vi "Graph (SubVI).vi"(9 "MeasChanel":u32[](array[numeric]), 10 "Parameters":T4={"UNDT_Type_signal"=enum."РЧ сигнал", "ФНЧ"=TRUE, "UNDT_Mean"=1, "IIR filter"={"Topology"=enum."Off", "Type"=enum."Bandpass", "Order"=4, "Lower Fc"=200000.0, "Upper Fc"=10000000.0, "PB Ripple"=1.0, "SB Attenuation"=60.0}, "ZeroDimension"=4000, "ТипДетектора"=enum."Оконный детектор", "FilterCor"={"HPFFilterNum"=enum."HPF_OFF", "LPFBode"=[], "HPFBode"=[], "EnableFilterСorrect"=FALSE, "LPF_Filter"=enum."14 МГц"}, "MeasControl"={"approx freq"=-1.0, "search (+/- % of Fsampl.)"=1.0, "start, duration"={"start samples/time"=-1.0, "duration"=0.0, "EnableSubset"=FALSE}, "averaging type"=enum."Linear", "window"=enum."Rectangular (none)", "hysteresis"=0.0, "level"=0.0}} {"MeasControl"."level" format="%.2p"; "MeasControl"."hysteresis" format="%.2p"; "MeasControl"."start, duration"."duration" format="%0.2f"; "MeasControl"."start, duration"."start samples/time" format="%0.2f"; "MeasControl"."search (+/- % of Fsampl.)" format="%#_13g"; "IIR filter"."PB Ripple" format="%0.2f"; "IIR filter"."SB Attenuation" format="%0.2f"; "IIR filter"."Lower Fc" format="%0.2p"; "IIR filter"."Upper Fc" format="%0.2p"; "UNDT_Mean" min=0 max=32 step=4}, 11 "DataIn":T1 {"UNDT_Cluster"."Gain Coeff" format="%#_6e"; "UNDT_Cluster"."Reserve 1" format="%02x"; "UNDT_Cluster"."Mux TX/RX" format="%02x"; "UNDT_Cluster"."ScanDelay" format="%02x"; "UNDT_Cluster"."PacketCounter" format="%08x"; "UNDT_Cluster"."SamplingInterval" format="%#_6e"; "UNDT_Cluster"."Lose Packet" format="%08x"; "UNDT_Cluster"."EncodersParam2" format="%016x"; "UNDT_Cluster"."EncodersParam1" format="%016x"; "UNDT_Cluster"."CRC 8" format="%02x"; "UNDT_Cluster"."N chanel" format="%02x"; "UNDT_Cluster"."N tick" format="%02x"; "UNDT_Cluster"."Ncycle" format="%04x"; "UNDT_Cluster"."FrameFormatVersion" format="%02x"; "UNDT_Cluster"."MagicWord" format="%.0x"}) -> (2 "Meas":T3 {"FFT amplitude mean" format="%.2p"; "DC" format="%0.2p"; "time trig 2" format="%0.2p"; "time trig" format="%0.2p"; "detected frequency 2" format="%.2p"; "way sensor 2" format="%.2p"; "way sensor 1" format="%.2p"; "detected frequency" format="%.2p"; "RMS" format="%0.2p"; "amplitude" format="%.2p"; "FFT amplitude" format="%.2p"}, 3 "Filtered X":dbl[](array[numeric]))   [LabVIEW 2017]
uses:
  Control_EU/UNDT_Graph (Type).ctl
  Control_EU/MeasControl2.ctl
  Control_EU/MeasControl.ctl
  Control_EU/DataCluster.ctl
  Control_EU/UNDT_ClusterPackRevers (Type).ctl
  <vilib>/Analysis/baseanly.llb/Mean (DBL).vi
  <vilib>/Analysis/NI_AALBase.lvlib
panel:
  out "Boolean":bool
  out "N tick":u8
  out "detected frequency":dbl
  out "FilterCorCoef":dbl
  out "MeanSizeLast":i32=8
  out "Tick 63":dbl[][](array[numeric])
  out "Tick 62":dbl[][](array[numeric])
  out "Tick 61":dbl[][](array[numeric])
  out "Tick 60":dbl[][](array[numeric])
  out "Tick 59":dbl[][](array[numeric])
  out "Tick 58":dbl[][](array[numeric])
  out "Tick 57":dbl[][](array[numeric])
  out "Tick 56":dbl[][](array[numeric])
  out "Tick 55":dbl[][](array[numeric])
  out "Tick 54":dbl[][](array[numeric])
  out "Tick 53":dbl[][](array[numeric])
  out "Tick 52":dbl[][](array[numeric])
  out "Tick 51":dbl[][](array[numeric])
  out "Tick 50":dbl[][](array[numeric])
  out "Tick 49":dbl[][](array[numeric])
  out "Tick 48":dbl[][](array[numeric])
  out "Tick 47":dbl[][](array[numeric])
  out "Tick 46":dbl[][](array[numeric])
  out "Tick 45":dbl[][](array[numeric])
  out "Tick 44":dbl[][](array[numeric])
  out "Tick 43":dbl[][](array[numeric])
  out "Tick 42":dbl[][](array[numeric])
  out "Tick 41":dbl[][](array[numeric])
  out "Tick 40":dbl[][](array[numeric])
  out "Tick 39":dbl[][](array[numeric])
  out "Tick 38":dbl[][](array[numeric])
  out "Tick 37":dbl[][](array[numeric])
  out "Tick 36":dbl[][](array[numeric])
  out "Tick 35":dbl[][](array[numeric])
  out "Tick 34":dbl[][](array[numeric])
  out "Tick 33":dbl[][](array[numeric])
  out "Tick 32":dbl[][](array[numeric])
  out "Tick 31":dbl[][](array[numeric])
  out "Tick 30":dbl[][](array[numeric])
  out "Tick 29":dbl[][](array[numeric])
  out "Tick 28":dbl[][](array[numeric])
  out "Tick 27":dbl[][](array[numeric])
  out "Tick 26":dbl[][](array[numeric])
  out "Tick 25":dbl[][](array[numeric])
  out "Tick 24":dbl[][](array[numeric])
  out "Tick 23":dbl[][](array[numeric])
  out "Tick 22":dbl[][](array[numeric])
  out "Tick 21":dbl[][](array[numeric])
  out "Tick 20":dbl[][](array[numeric])
  out "Tick 19":dbl[][](array[numeric])
  out "Tick 18":dbl[][](array[numeric])
  out "Tick 17":dbl[][](array[numeric])
  out "Tick 16":dbl[][](array[numeric])
  out "Tick 15":dbl[][](array[numeric])
  out "Tick 14":dbl[][](array[numeric])
  out "Tick 13":dbl[][](array[numeric])
  out "Tick 12":dbl[][](array[numeric])
  out "Tick 11":dbl[][](array[numeric])
  out "Tick 10":dbl[][](array[numeric])
  out "Tick 9":dbl[][](array[numeric])
  out "Tick 8":dbl[][](array[numeric])
  out "Tick 7":dbl[][](array[numeric])
  out "Tick 6":dbl[][](array[numeric])
  out "Tick 5":dbl[][](array[numeric])
  out "Tick 4":dbl[][](array[numeric])
  out "Tick 3":dbl[][](array[numeric])
  out "Tick 2":dbl[][](array[numeric])
  out "Tick 1":dbl[][](array[numeric])
  out "Tick 0":dbl[][](array[numeric])
  out "MeanSize":i32=8
  out "Index Aarray":i32[](array[numeric])
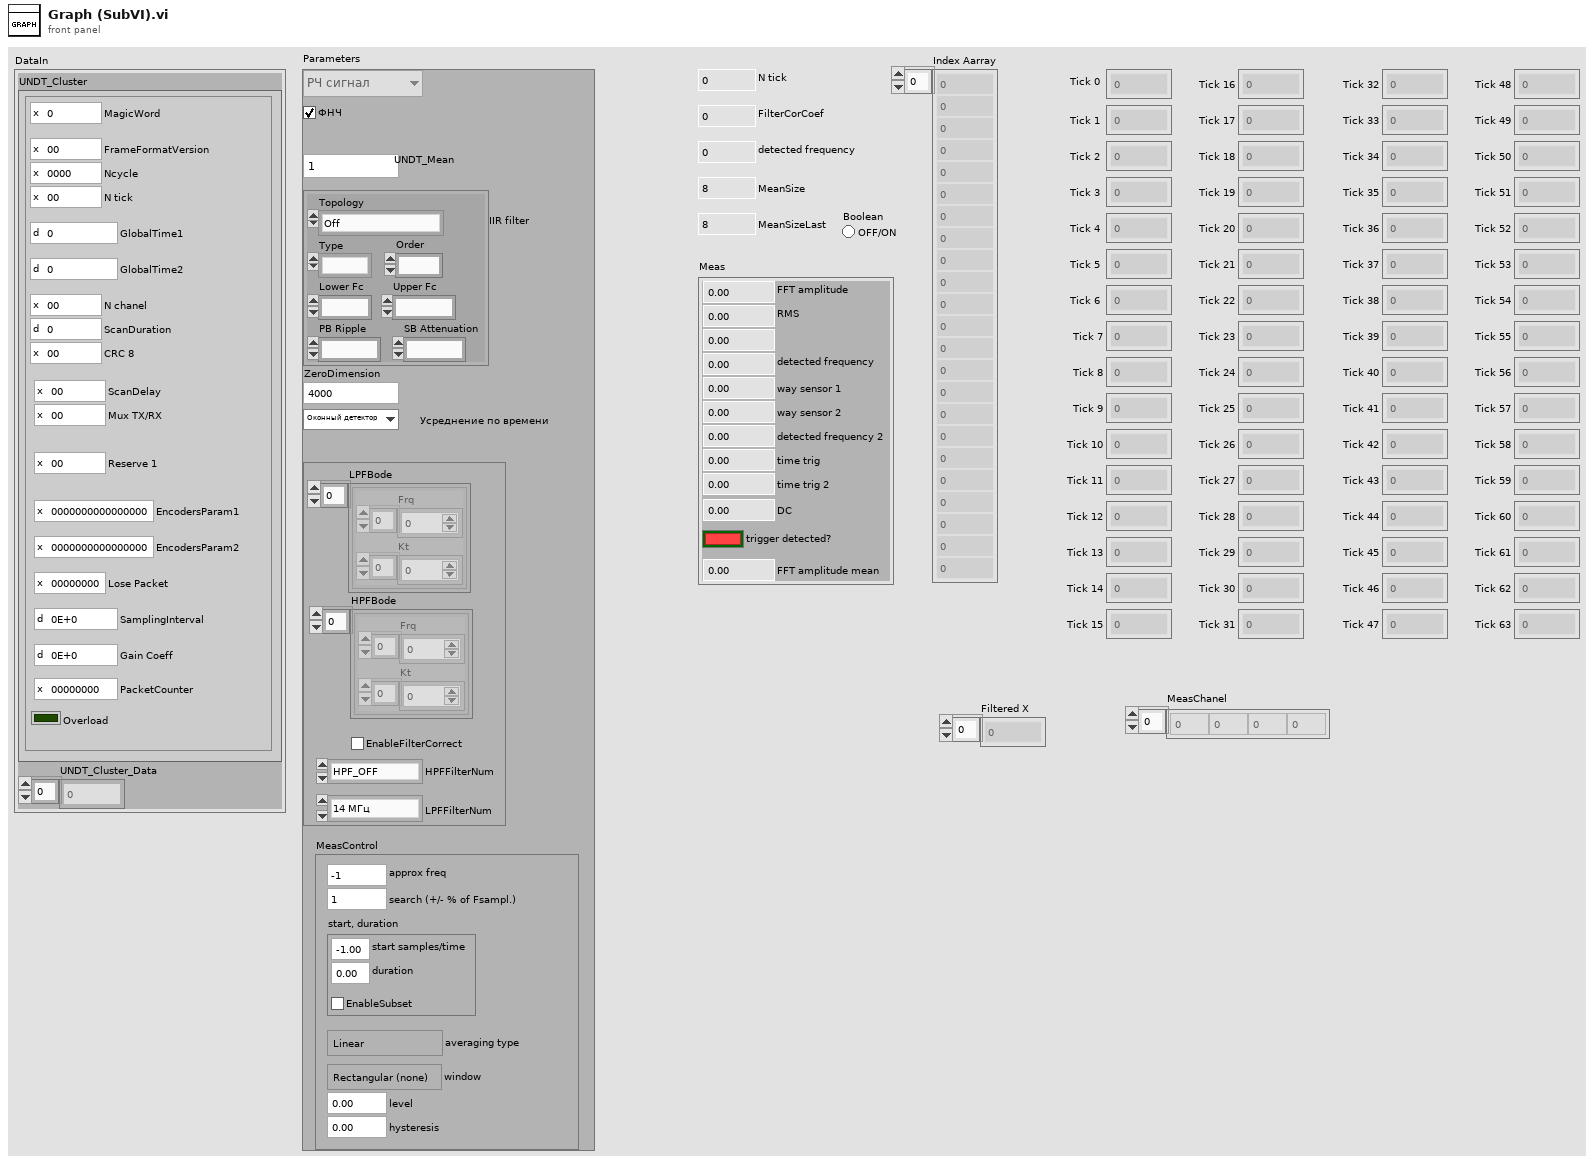
[diagram p1: front panel]
types:
  T1 = typedef "DataCluster.ctl" = cluster{"UNDT_Cluster":T2, "UNDT_Cluster_Data":dbl[]}
  T2 = typedef "UNDT_ClusterPackRevers (Type).ctl" = cluster{"PacketCounter":u32, "Gain Coeff":sgl, "SamplingInterval":sgl, "Lose Packet":u32, "EncodersParam2":u64, "EncodersParam1":u64, "Reserve 1":u8, "Mux TX/RX":u8, "ScanDelay":u16, "CRC 8":u8, "ScanDuration":u16, "N chanel":u8, "GlobalTime2":u32, "GlobalTime1":u32, "N tick":u8, "Ncycle":u16, "FrameFormatVersion":u8, "MagicWord":u32, "Overload":bool}
  T3 = typedef "MeasControl.ctl" = cluster{"FFT amplitude":dbl, "amplitude":dbl, "RMS":dbl, "detected frequency":dbl, "way sensor 1":ext, "way sensor 2":ext, "detected frequency 2":dbl, "time trig":dbl, "time trig 2":dbl, "DC":dbl, "trigger detected?":bool, "FFT amplitude mean":dbl}
  T4 = typedef "UNDT_Graph (Type).ctl" = cluster{"UNDT_Type_signal":enum16{"РЧ сигнал", "Детект. полное", "Положит.", "Отрицат."}, "ФНЧ":bool, "UNDT_Mean":i32, "IIR filter":cluster{"Topology":enum16{"Off", "Butterworth", "Chebyshev", "Inverse Chebyshev", "Elliptic", "Bessel"}, "Type":enum16{"Lowpass", "Highpass", "Bandpass", "Bandstop"}, "Order":i32, "Lower Fc":dbl, "Upper Fc":dbl, "PB Ripple":dbl, "SB Attenuation":dbl}, "ZeroDimension":i32, "ТипДетектора":enum16{"Оконный детектор", "Гильберт"}, "FilterCor":cluster{"HPFFilterNum":enum16{"HPF_OFF", "1", "2", "3", "4", "5", "6", "7", "8", "9", "10"}, "LPFBode":cluster{"Frq":dbl[], "Kt":dbl[]}[], "HPFBode":cluster{"Frq":dbl[], "Kt":dbl[]}[], "EnableFilterСorrect":bool, "LPF_Filter":enum16{"14 МГц", "10 МГц", "7.5 МГц", "Выкл."}}, "MeasControl":T5}
  T5 = typedef "MeasControl2.ctl" = cluster{"approx freq":dbl, "search (+/- % of Fsampl.)":dbl, "start, duration":cluster{"start samples/time":dbl, "duration":dbl, "EnableSubset":bool}, "averaging type":enum16{"Linear", "Exponential"}, "window":enum16{"Rectangular (none)", "Hanning", "Low side lobe"}, "hysteresis":dbl, "level":dbl}
  T6 = enum16{"РЧ сигнал", "Детект. полное", "Положит.", "Отрицат."}
  T7 = cluster{"Topology":enum16{"Off", "Butterworth", "Chebyshev", "Inverse Chebyshev", "Elliptic", "Bessel"}, "Type":enum16{"Lowpass", "Highpass", "Bandpass", "Bandstop"}, "Order":i32, "Lower Fc":dbl, "Upper Fc":dbl, "PB Ripple":dbl, "SB Attenuation":dbl}
  T8 = cluster{"HPFFilterNum":enum16{"HPF_OFF", "1", "2", "3", "4", "5", "6", "7", "8", "9", "10"}, "LPFBode":cluster{"Frq":dbl[], "Kt":dbl[]}[], "HPFBode":cluster{"Frq":dbl[], "Kt":dbl[]}[], "EnableFilterСorrect":bool, "LPF_Filter":enum16{"14 МГц", "10 МГц", "7.5 МГц", "Выкл."}}
  T9 = enum16{"HPF_OFF", "1", "2", "3", "4", "5", "6", "7", "8", "9", "10"}
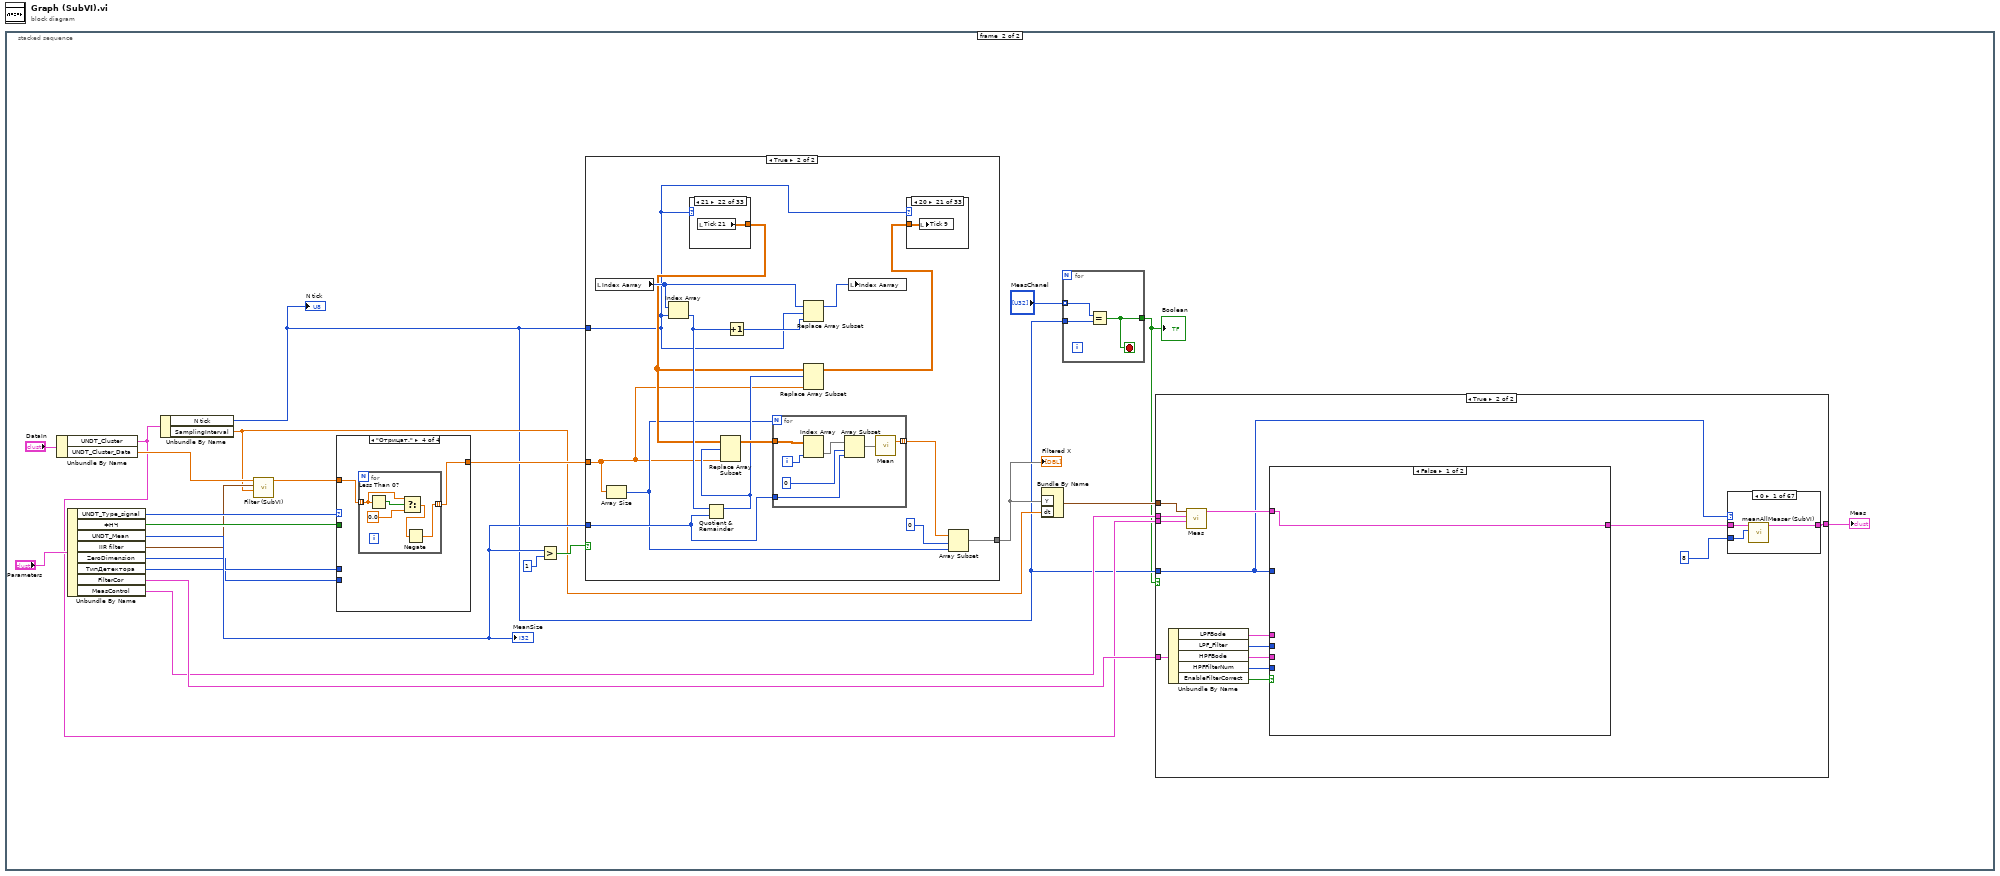
[diagram p0: block diagram]
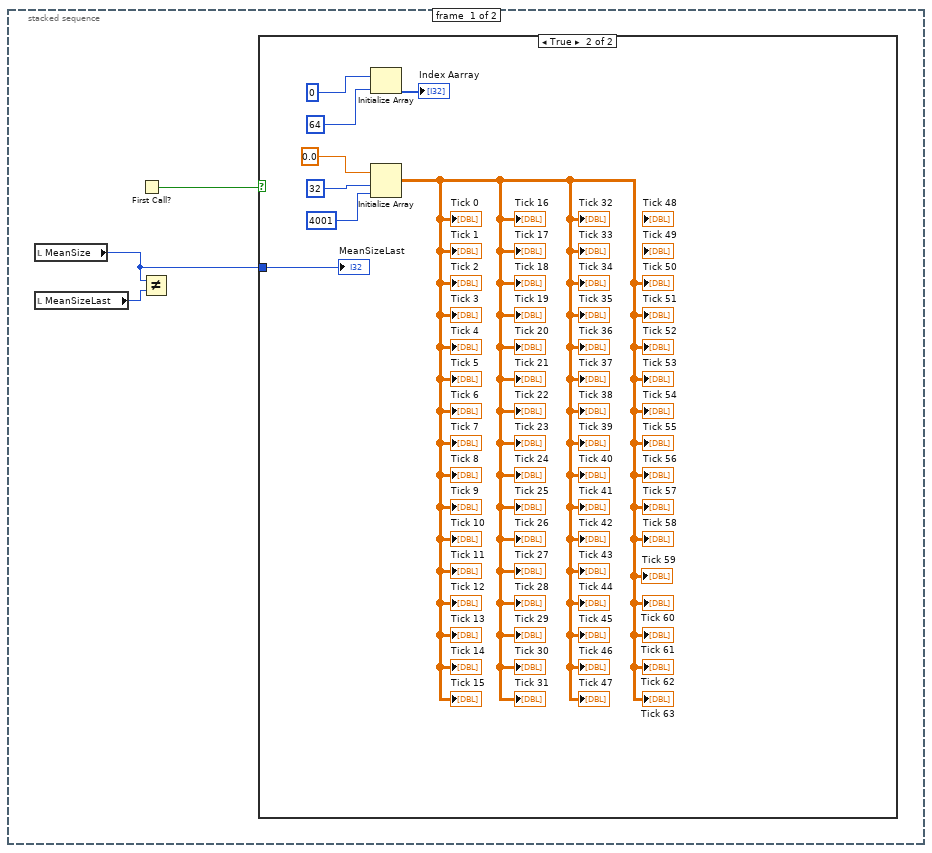
[diagram p2: hidden frame]
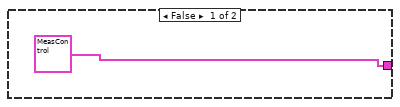
[diagram p4: hidden frame]
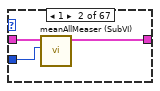
[diagram p5: hidden frame]
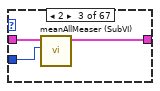
[diagram p6: hidden frame]
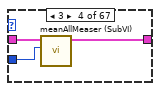
[diagram p7: hidden frame]
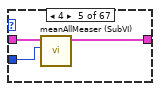
[diagram p8: hidden frame]
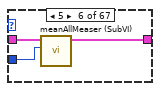
[diagram p9: hidden frame]
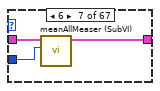
[diagram p10: hidden frame]
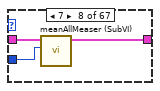
[diagram p11: hidden frame]
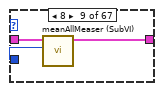
[diagram p12: hidden frame]
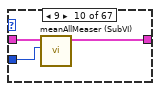
[diagram p13: hidden frame]
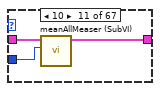
[diagram p14: hidden frame]
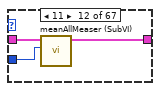
[diagram p15: hidden frame]
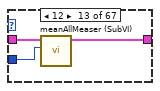
[diagram p16: hidden frame]
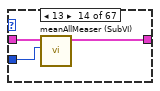
[diagram p17: hidden frame]
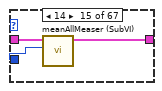
[diagram p18: hidden frame]
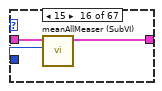
[diagram p19: hidden frame]
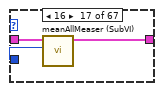
[diagram p20: hidden frame]
diagram:
  n1 = stacked-sequence {
    frame #0 {
      n2 = local read "MeanSize"() -> (w1:i32)
      n3 = local read "MeanSizeLast"() -> (w3:i32)
      n4 = First Call?() -> (First Call?: T/F=w2:bool)
      n5 = Not Equal?(x=w1, y=w3) -> ()  [unwired: 1 out]
      n6 = case shown="True" w2 {
        tunnel: w1 -> [_ w6]
        frame False {
        }
        frame True {
          n7 = Initialize Array(0 ("element"), 64 ("dimension size")) -> (→"Index Aarray":i32[])
          n8 = Initialize Array(0.0 ("element"), 32 ("dimension size"), 4001 ("dimension size")) -> (→"Tick 0" →"Tick 1" →"Tick 2" →"Tick 3" →"Tick 4" →"Tick 5" →"Tick 6" →"Tick 7" →"Tick 8" →"Tick 9" →"Tick 10" →"Tick 11" →"Tick 12" →"Tick 13" →"Tick 14" →"Tick 15" →"Tick 16" →"Tick 33" →"Tick 32" →"Tick 31" →"Tick 30" →"Tick 29" →"Tick 28" →"Tick 27" →"Tick 26" →"Tick 25" →"Tick 24" →"Tick 23" →"Tick 22" →"Tick 21" →"Tick 20" →"Tick 19" →"Tick 18" →"Tick 17" →"Tick 50" →"Tick 47" →"Tick 46" →"Tick 45" →"Tick 44" →"Tick 43" →"Tick 42" →"Tick 41" →"Tick 40" →"Tick 39" →"Tick 38" →"Tick 37" →"Tick 36" →"Tick 35" →"Tick 34" →"Tick 63" →"Tick 62" →"Tick 61" →"Tick 60" →"Tick 59" →"Tick 58" →"Tick 57" →"Tick 56" →"Tick 55" →"Tick 54" →"Tick 53" →"Tick 52" →"Tick 51":dbl[][])
          "MeanSizeLast" <- w6
        }
      }
    }
    frame #1 {
      n9 = Unbundle By Name("DataIn") -> ("UNDT_Cluster"=w16:T2, "UNDT_Cluster_Data"=w23:dbl[])
      n10 = Unbundle By Name("Parameters") -> ("UNDT_Type_signal"=w33:T6, "ФНЧ"=w32:bool, "UNDT_Mean"=w28:i32, "IIR filter"=w22:T7, "ZeroDimension"=w27:i32, "ТипДетектора"=w25:enum16{"Оконный детектор", "Гильберт"}, "FilterCor"=w24:T8, "MeasControl"=w18:T5)
      "MeanSize" <- w28
      n11 = Unbundle By Name(w16) -> ("N tick"=w13:u8, "SamplingInterval"=w21:sgl)
      "N tick" <- w13
      n12 = call "Filter (SubVI).vi"("SamplingInterval"=w21, "IIR filter"=w22, "UNDT_Cluster_Data"=w23) -> ("Filtered X"=w19:dbl[])  [unwired: 8 in]
      n13 = case shown="\"Отрицат.\"" w33 {
        tunnel: w19 -> [w359 w362 w374 w380]
        tunnel: [w359 w364 w373 w379] -> w31
        tunnel: w32 -> [_ w363 _ _]
        tunnel: w27 -> [_ w361 _ _]
        tunnel: w25 -> [_ w360 _ _]
        frame "РЧ сигнал", Default {
        }
        frame "Детект. полное" {
          n14 = case shown="\"Оконный детектор\", Default" w360 {
            tunnel: [w367 w372] -> w364
            tunnel: w363 -> [w366 w371]
            tunnel: w362 -> [w368 w370]
            tunnel: w361 -> [w365 w369]
            frame "Оконный детектор", Default {
              n15 = call "Detect (SubVI).vi"("Фильтр"=w366, "Array in"=w368, "length"=w365) -> ("Array out"=w367:dbl[])  [unwired: 8 in]
            }
            frame "Гильберт" {
              n16 = call "LPF (SubVI).vi"("ZeroDimension"=w369, "ФНЧ"=w371, "In"=w370) -> ("Filtered X"=w372:dbl[])  [unwired: 8 in]
            }
          }
        }
        frame "Положит." {
          n17 = for {
            tunnel: w374 -> [w377] mode=indexing
            tunnel: [w375] -> w373 mode=indexing
            n18 = Greater Than 0?(x=w377) -> (x > 0?=w378:bool)
            n19 = Select(t=w377, s=w378, f=0.0) -> (s? t:f=w375:dbl)
          }
        }
        frame "Отрицат." {
          n20 = for {
            tunnel: w380 -> [w384] mode=indexing
            tunnel: [w381] -> w379 mode=indexing
            n21 = Less Than 0?(x=w384) -> (x < 0?=w385:bool)
            n22 = Select(t=w384, s=w385, f=0.0) -> (s? t:f=w382:dbl)
            n23 = Negate(x=w382) -> (-x=w381:dbl)
          }
        }
      }
      n24 = Greater?(x=w28, y=1) -> (0:w29:bool)
      n25 = case shown="True" w29 {
        tunnel: w31 -> [w270 w271]
        tunnel: [w270 w283] -> w17
        tunnel: w13 -> [_ w276]
        tunnel: w28 -> [_ w273]
        frame False {
        }
        frame True {
          n26 = local read "Index Aarray"() -> (w280:i32[])
          n27 = Array Size(array=w271) -> (size(s)=w272:i32)
          n28 = Index Array(array=w280, index=w276) -> (element=w279:i32)
          n29 = case shown="21" w276 {
            tunnel: [w319 w320 w321 w322 w323 w324 w325 w326 w327 w328 w329 w330 w331 w332 w333 w334 w335 w336 w337 w338 w339 w340 w341 w342 w343 w344 w345 w346 w347 w348 w349 w350 w351] -> w277
            frame 0 {
              n30 = local read "Tick 0"() -> (w319:dbl[][])
            }
            frame 1 {
              n31 = local read "Tick 1"() -> (w320:dbl[][])
            }
            frame 2, Default {
              n32 = local read "Tick 2"() -> (w321:dbl[][])
            }
            frame 3 {
              n33 = local read "Tick 3"() -> (w322:dbl[][])
            }
            frame 4 {
              n34 = local read "Tick 4"() -> (w323:dbl[][])
            }
            frame 5 {
              n35 = local read "Tick 5"() -> (w324:dbl[][])
            }
            frame 6 {
              n36 = local read "Tick 6"() -> (w325:dbl[][])
            }
            frame 7 {
              n37 = local read "Tick 7"() -> (w326:dbl[][])
            }
            frame 8 {
              n38 = local read "Tick 8"() -> (w327:dbl[][])
            }
            frame 9 {
              n39 = local read "Tick 9"() -> (w328:dbl[][])
            }
            frame 10 {
              n40 = local read "Tick 10"() -> (w329:dbl[][])
            }
            frame 11 {
              n41 = local read "Tick 11"() -> (w330:dbl[][])
            }
            frame 12 {
              n42 = local read "Tick 12"() -> (w331:dbl[][])
            }
            frame 13 {
              n43 = local read "Tick 13"() -> (w332:dbl[][])
            }
            frame 14 {
              n44 = local read "Tick 14"() -> (w333:dbl[][])
            }
            frame 15 {
              n45 = local read "Tick 15"() -> (w334:dbl[][])
            }
            frame 16 {
              n46 = local read "Tick 16"() -> (w335:dbl[][])
            }
            frame 17 {
              n47 = local read "Tick 17"() -> (w336:dbl[][])
            }
            frame 18 {
              n48 = local read "Tick 18"() -> (w337:dbl[][])
            }
            frame 19 {
              n49 = local read "Tick 19"() -> (w338:dbl[][])
            }
            frame 20 {
              n50 = local read "Tick 20"() -> (w339:dbl[][])
            }
            frame 21 {
              n51 = local read "Tick 21"() -> (w340:dbl[][])
            }
            frame 22 {
              n52 = local read "Tick 22"() -> (w341:dbl[][])
            }
            frame 23 {
              n53 = local read "Tick 23"() -> (w342:dbl[][])
            }
            frame 24 {
              n54 = local read "Tick 24"() -> (w343:dbl[][])
            }
            frame 25 {
              n55 = local read "Tick 25"() -> (w344:dbl[][])
            }
            frame 26 {
              n56 = local read "Tick 26"() -> (w345:dbl[][])
            }
            frame 27 {
              n57 = local read "Tick 27"() -> (w346:dbl[][])
            }
            frame 28 {
              n58 = local read "Tick 28"() -> (w347:dbl[][])
            }
            frame 29 {
              n59 = local read "Tick 29"() -> (w348:dbl[][])
            }
            frame 30 {
              n60 = local read "Tick 30"() -> (w349:dbl[][])
            }
            frame 31 {
              n61 = local read "Tick 31"() -> (w350:dbl[][])
            }
            frame 32 {
              n62 = local read "Tick 32"() -> (w351:dbl[][])
            }
          }
          n63 = Quotient & Remainder(x=w279, y=w273) -> (x-y*floor(x/y)=w274:i32)  [unwired: 1 out]
          n64 = Replace Array Subset(array=w277, new element=w271, index (row)=w274) -> (w285:dbl[][])  [unwired: 1 in]
          n65 = Increment(x=w279) -> (x+1=w281:i32)
          n66 = for {
            N: w272 -> [_]
            tunnel: w285 -> [w357]
            tunnel: [w358] -> w278 mode=indexing
            tunnel: w273 -> [w353]
            i -> [w356]
            n67 = Index Array(array=w357, index (col)=w356) -> (element=w355:dbl[])  [unwired: 1 in]
            n68 = Array Subset(array=w355, index=0, length=w353) -> (w352:dbl[])
            n69 = call-poly <vilib>:"Mean.vi"("X"=w352) -> ("mean"=w358:dbl)  [unwired: 1 out]
          }
          n70 = Replace Array Subset(array=w280, new element=w281, index=w276) -> (w282:i32[])
          n71 = Replace Array Subset(array=w277, new element=w271, index (row)=w274) -> (w275:dbl[][])  [unwired: 1 in]
          n72 = local write "Index Aarray"(w282) -> ()
          n73 = case shown="20" w276 {
            tunnel: w275 -> [w286 w287 w288 w289 w290 w291 w292 w293 w294 w295 w296 w297 w298 w299 w300 w301 w302 w303 w304 w305 w306 w307 w308 w309 w310 w311 w312 w313 w314 w315 w316 w317 w318]
            frame 0 {
              n74 = local write "Tick 0"(w286) -> ()
            }
            frame 1 {
              n75 = local write "Tick 1"(w287) -> ()
            }
            frame 2, Default {
              n76 = local write "Tick 2"(w288) -> ()
            }
            frame 3 {
              n77 = local write "Tick 3"(w289) -> ()
            }
            frame 4 {
              n78 = local write "Tick 4"(w290) -> ()
            }
            frame 5 {
              n79 = local write "Tick 5"(w291) -> ()
            }
            frame 6 {
              n80 = local write "Tick 6"(w292) -> ()
            }
            frame 7 {
              n81 = local write "Tick 7"(w293) -> ()
            }
            frame 8 {
              n82 = local write "Tick 8"(w294) -> ()
            }
            frame 9 {
              n83 = local write "Tick 9"(w295) -> ()
            }
            frame 10 {
              n84 = local write "Tick 9"(w296) -> ()
            }
            frame 11 {
              n85 = local write "Tick 9"(w297) -> ()
            }
            frame 12 {
              n86 = local write "Tick 9"(w298) -> ()
            }
            frame 13 {
              n87 = local write "Tick 9"(w299) -> ()
            }
            frame 14 {
              n88 = local write "Tick 9"(w300) -> ()
            }
            frame 15 {
              n89 = local write "Tick 9"(w301) -> ()
            }
            frame 16 {
              n90 = local write "Tick 9"(w302) -> ()
            }
            frame 17 {
              n91 = local write "Tick 9"(w303) -> ()
            }
            frame 18 {
              n92 = local write "Tick 9"(w304) -> ()
            }
            frame 19 {
              n93 = local write "Tick 9"(w305) -> ()
            }
            frame 20 {
              n94 = local write "Tick 9"(w306) -> ()
            }
            frame 21 {
              n95 = local write "Tick 9"(w307) -> ()
            }
            frame 22 {
              n96 = local write "Tick 9"(w308) -> ()
            }
            frame 23 {
              n97 = local write "Tick 9"(w309) -> ()
            }
            frame 24 {
              n98 = local write "Tick 9"(w310) -> ()
            }
            frame 25 {
              n99 = local write "Tick 9"(w311) -> ()
            }
            frame 26 {
              n100 = local write "Tick 9"(w312) -> ()
            }
            frame 27 {
              n101 = local write "Tick 9"(w313) -> ()
            }
            frame 28 {
              n102 = local write "Tick 9"(w314) -> ()
            }
            frame 29 {
              n103 = local write "Tick 9"(w315) -> ()
            }
            frame 30 {
              n104 = local write "Tick 9"(w316) -> ()
            }
            frame 31 {
              n105 = local write "Tick 9"(w317) -> ()
            }
            frame 32 {
              n106 = local write "Tick 32"(w318) -> ()
            }
          }
          n107 = Array Subset(array=w278, index=0, length=w272) -> (w283:dbl[])
        }
      }
      "Filtered X" <- w17
      n108 = Bundle By Name("Y"=w17, "dt"=w21) -> (w26:waveform(dbl))  [unwired: 1 in]
      n109 = for {
        tunnel: "MeasChanel" -> [w268] mode=indexing
        tunnel: w13 -> [w269]
        tunnel: [w267] -> w12
        stop <- w267 stop-if-true
        n110 = Equal?(x=w268, y=w269) -> (x = y?=w267:bool)
      }
      "Boolean" <- w12
      n111 = case shown="True" w12 {
        tunnel: w26 -> [_ w43]
        tunnel: w24 -> [_ w42]
        tunnel: w18 -> [_ w41]
        tunnel: w16 -> [_ w40]
        tunnel: [T3 {"FFT amplitude"=nan, "amplitude"=nan, "RMS"=nan, "detected frequency"=nan, "way sensor 1"=0.0, "way sensor 2"=0.0, "detected frequency 2"=0.0, "time trig"=0.0, "time trig 2"=0.0, "DC"=0.0, "trigger detected?"=FALSE, "FFT amplitude mean"=0.0} ("Meas") w37] -> w15
        tunnel: w13 -> [_ w36]
        frame False {
        }
        frame True {
          n112 = Unbundle By Name(w42) -> ("LPFBode"=w47:cluster{"Frq":dbl[], "Kt":dbl[]}[], "LPF_Filter"=w46:enum16{"14 МГц", "10 МГц", "7.5 МГц", "Выкл."}, "HPFBode"=w45:cluster{"Frq":dbl[], "Kt":dbl[]}[], "HPFFilterNum"=w44:T9, "EnableFilterСorrect"=w48:bool)
          n113 = call "Meas.vi"("input cluster"=w40, "MeasControl"=w41, "signal_in"=w43) -> ("Meas"=w49:T3)  [unwired: 8 in]
          n114 = case shown="False" w48 {
            tunnel: w49 -> [w251 w263]
            tunnel: [w251 w262] -> w38
            tunnel: w47 -> [_ w260]
            tunnel: w46 -> [_ w259]
            tunnel: w45 -> [_ w258]
            tunnel: w44 -> [_ w257]
            tunnel: w36 -> [_ w252]
            frame False {
            }
            frame True {
              n115 = Unbundle By Name(w263) -> ("FFT amplitude"=w264:dbl, "amplitude"=w266:dbl, "RMS"=w265:dbl, "detected frequency"=w261:dbl)
              "detected frequency" <- w261
              n116 = call "KtFilter (SubVI).vi"("N tick"=w252, "frq"=w261, "LPF_Filter"=w259, "Array"=w260) -> ("Numeric"=w253:dbl)  [unwired: 7 in]
              "FilterCorCoef" <- w253
              n117 = call "KtFilterHPF (SubVI).vi"("frq"=w261, "HPFFilterNum"=w257, "Array"=w258) -> ()  [unwired: 8 in, 1 out]
              n118 = Divide(x=w265, y=w253) -> (x/y=w254:dbl)
              n119 = Divide(x=w264, y=w253) -> (x/y=w256:dbl)
              n120 = Divide(x=w266, y=w253) -> (x/y=w255:dbl)
              n121 = Bundle By Name(cluster=w263, "FFT amplitude"=w256, "amplitude"=w255, "RMS"=w254) -> (w262:T3)
            }
          }
          n122 = case shown="0" w36 {
            tunnel: w38 -> [w51 w55 w58 w61 w64 w67 w70 w73 w76 w79 w82 w85 w88 w91 w94 w97 w100 w103 w106 w109 w112 w115 w118 w121 w124 w127 w130 w133 w136 w139 w142 w145 w147 w151 w154 w157 w160 w163 w166 w169 w172 w175 w178 w181 w184 w187 w190 w193 w196 w199 w202 w205 w208 w211 w214 w217 w220 w223 w226 w229 w232 w235 w238 w241 w244 w247 w250]
            tunnel: [w50 w53 w57 w60 w63 w66 w69 w72 w75 w78 w81 w84 w87 w90 w93 w96 w99 w102 w105 w108 w111 w114 w117 w120 w123 w126 w129 w132 w135 w138 w141 w144 w146 w150 w153 w156 w159 w162 w165 w168 w171 w174 w177 w180 w183 w186 w189 w192 w195 w198 w201 w204 w207 w210 w213 w216 w219 w222 w225 w228 w231 w234 w237 w240 w243 w246 w249] -> w37
            tunnel: 8 ("mMean") -> [w52 w54 w56 w59 w62 w65 w68 w71 w74 w77 w80 w83 w86 w89 w92 w95 w98 w101 w104 w107 w110 w113 w116 w119 w122 w125 w128 w131 w134 w137 w140 w143 w148 w149 w152 w155 w158 w161 w164 w167 w170 w173 w176 w179 w182 w185 w188 w191 w194 w197 w200 w203 w206 w209 w212 w215 w218 w221 w224 w227 w230 w233 w236 w239 w242 w245 w248]
            frame 0 {
              n123 = call "meanAllMeaser (SubVI).vi"("mMean"=w52, "MeasIn"=w51) -> ("MeasOut"=w50:T3)  [unwired: 9 in]
            }
            frame 1 {
              n124 = call "meanAllMeaser (SubVI).vi"("mMean"=w54, "MeasIn"=w55) -> ("MeasOut"=w53:T3)  [unwired: 9 in]
            }
            frame 2 {
              n125 = call "meanAllMeaser (SubVI).vi"("mMean"=w56, "MeasIn"=w58) -> ("MeasOut"=w57:T3)  [unwired: 9 in]
            }
            frame 3 {
              n126 = call "meanAllMeaser (SubVI).vi"("mMean"=w59, "MeasIn"=w61) -> ("MeasOut"=w60:T3)  [unwired: 9 in]
            }
            frame 4 {
              n127 = call "meanAllMeaser (SubVI).vi"("mMean"=w62, "MeasIn"=w64) -> ("MeasOut"=w63:T3)  [unwired: 9 in]
            }
            frame 5 {
              n128 = call "meanAllMeaser (SubVI).vi"("mMean"=w65, "MeasIn"=w67) -> ("MeasOut"=w66:T3)  [unwired: 9 in]
            }
            frame 6 {
              n129 = call "meanAllMeaser (SubVI).vi"("mMean"=w68, "MeasIn"=w70) -> ("MeasOut"=w69:T3)  [unwired: 9 in]
            }
            frame 7 {
              n130 = call "meanAllMeaser (SubVI).vi"("mMean"=w71, "MeasIn"=w73) -> ("MeasOut"=w72:T3)  [unwired: 9 in]
            }
            frame 8 {
              n131 = call "meanAllMeaser (SubVI).vi"("mMean"=w74, "MeasIn"=w76) -> ("MeasOut"=w75:T3)  [unwired: 9 in]
            }
            frame 9 {
              n132 = call "meanAllMeaser (SubVI).vi"("mMean"=w77, "MeasIn"=w79) -> ("MeasOut"=w78:T3)  [unwired: 9 in]
            }
            frame 10 {
              n133 = call "meanAllMeaser (SubVI).vi"("mMean"=w80, "MeasIn"=w82) -> ("MeasOut"=w81:T3)  [unwired: 9 in]
            }
            frame 11 {
              n134 = call "meanAllMeaser (SubVI).vi"("mMean"=w83, "MeasIn"=w85) -> ("MeasOut"=w84:T3)  [unwired: 9 in]
            }
            frame 12 {
              n135 = call "meanAllMeaser (SubVI).vi"("mMean"=w86, "MeasIn"=w88) -> ("MeasOut"=w87:T3)  [unwired: 9 in]
            }
            frame 13 {
              n136 = call "meanAllMeaser (SubVI).vi"("mMean"=w89, "MeasIn"=w91) -> ("MeasOut"=w90:T3)  [unwired: 9 in]
            }
            frame 14 {
              n137 = call "meanAllMeaser (SubVI).vi"("mMean"=w92, "MeasIn"=w94) -> ("MeasOut"=w93:T3)  [unwired: 9 in]
            }
            frame 15 {
              n138 = call "meanAllMeaser (SubVI).vi"("mMean"=w95, "MeasIn"=w97) -> ("MeasOut"=w96:T3)  [unwired: 9 in]
            }
            frame 16 {
              n139 = call "meanAllMeaser (SubVI).vi"("mMean"=w98, "MeasIn"=w100) -> ("MeasOut"=w99:T3)  [unwired: 9 in]
            }
            frame 17 {
              n140 = call "meanAllMeaser (SubVI).vi"("mMean"=w101, "MeasIn"=w103) -> ("MeasOut"=w102:T3)  [unwired: 9 in]
            }
            frame 18 {
              n141 = call "meanAllMeaser (SubVI).vi"("mMean"=w104, "MeasIn"=w106) -> ("MeasOut"=w105:T3)  [unwired: 9 in]
            }
            frame 19 {
              n142 = call "meanAllMeaser (SubVI).vi"("mMean"=w107, "MeasIn"=w109) -> ("MeasOut"=w108:T3)  [unwired: 9 in]
            }
            frame 20 {
              n143 = call "meanAllMeaser (SubVI).vi"("mMean"=w110, "MeasIn"=w112) -> ("MeasOut"=w111:T3)  [unwired: 9 in]
            }
            frame 21 {
              n144 = call "meanAllMeaser (SubVI).vi"("mMean"=w113, "MeasIn"=w115) -> ("MeasOut"=w114:T3)  [unwired: 9 in]
            }
            frame 22 {
              n145 = call "meanAllMeaser (SubVI).vi"("mMean"=w116, "MeasIn"=w118) -> ("MeasOut"=w117:T3)  [unwired: 9 in]
            }
            frame 23 {
              n146 = call "meanAllMeaser (SubVI).vi"("mMean"=w119, "MeasIn"=w121) -> ("MeasOut"=w120:T3)  [unwired: 9 in]
            }
            frame 24 {
              n147 = call "meanAllMeaser (SubVI).vi"("mMean"=w122, "MeasIn"=w124) -> ("MeasOut"=w123:T3)  [unwired: 9 in]
            }
            frame 25 {
              n148 = call "meanAllMeaser (SubVI).vi"("mMean"=w125, "MeasIn"=w127) -> ("MeasOut"=w126:T3)  [unwired: 9 in]
            }
            frame 26 {
              n149 = call "meanAllMeaser (SubVI).vi"("mMean"=w128, "MeasIn"=w130) -> ("MeasOut"=w129:T3)  [unwired: 9 in]
            }
            frame 27 {
              n150 = call "meanAllMeaser (SubVI).vi"("mMean"=w131, "MeasIn"=w133) -> ("MeasOut"=w132:T3)  [unwired: 9 in]
            }
            frame 28 {
              n151 = call "meanAllMeaser (SubVI).vi"("mMean"=w134, "MeasIn"=w136) -> ("MeasOut"=w135:T3)  [unwired: 9 in]
            }
            frame 29 {
              n152 = call "meanAllMeaser (SubVI).vi"("mMean"=w137, "MeasIn"=w139) -> ("MeasOut"=w138:T3)  [unwired: 9 in]
            }
            frame 30 {
              n153 = call "meanAllMeaser (SubVI).vi"("mMean"=w140, "MeasIn"=w142) -> ("MeasOut"=w141:T3)  [unwired: 9 in]
            }
            frame 31 {
              n154 = call "meanAllMeaser (SubVI).vi"("mMean"=w143, "MeasIn"=w145) -> ("MeasOut"=w144:T3)  [unwired: 9 in]
            }
            frame 32 {
              n155 = call "meanAllMeaser (SubVI).vi"("mMean"=w148, "MeasIn"=w147) -> ("MeasOut"=w146:T3)  [unwired: 9 in]
            }
            frame 33 {
              n156 = call "meanAllMeaser (SubVI).vi"("mMean"=w149, "MeasIn"=w151) -> ("MeasOut"=w150:T3)  [unwired: 9 in]
            }
            frame 34 {
              n157 = call "meanAllMeaser (SubVI).vi"("mMean"=w152, "MeasIn"=w154) -> ("MeasOut"=w153:T3)  [unwired: 9 in]
            }
            frame 35 {
              n158 = call "meanAllMeaser (SubVI).vi"("mMean"=w155, "MeasIn"=w157) -> ("MeasOut"=w156:T3)  [unwired: 9 in]
            }
            frame 36 {
              n159 = call "meanAllMeaser (SubVI).vi"("mMean"=w158, "MeasIn"=w160) -> ("MeasOut"=w159:T3)  [unwired: 9 in]
            }
            frame 37 {
              n160 = call "meanAllMeaser (SubVI).vi"("mMean"=w161, "MeasIn"=w163) -> ("MeasOut"=w162:T3)  [unwired: 9 in]
            }
            frame 38 {
              n161 = call "meanAllMeaser (SubVI).vi"("mMean"=w164, "MeasIn"=w166) -> ("MeasOut"=w165:T3)  [unwired: 9 in]
            }
            frame 39 {
              n162 = call "meanAllMeaser (SubVI).vi"("mMean"=w167, "MeasIn"=w169) -> ("MeasOut"=w168:T3)  [unwired: 9 in]
            }
            frame 40 {
              n163 = call "meanAllMeaser (SubVI).vi"("mMean"=w170, "MeasIn"=w172) -> ("MeasOut"=w171:T3)  [unwired: 9 in]
            }
            frame 41 {
              n164 = call "meanAllMeaser (SubVI).vi"("mMean"=w173, "MeasIn"=w175) -> ("MeasOut"=w174:T3)  [unwired: 9 in]
            }
            frame 42 {
              n165 = call "meanAllMeaser (SubVI).vi"("mMean"=w176, "MeasIn"=w178) -> ("MeasOut"=w177:T3)  [unwired: 9 in]
            }
            frame 43 {
              n166 = call "meanAllMeaser (SubVI).vi"("mMean"=w179, "MeasIn"=w181) -> ("MeasOut"=w180:T3)  [unwired: 9 in]
            }
            frame 44 {
              n167 = call "meanAllMeaser (SubVI).vi"("mMean"=w182, "MeasIn"=w184) -> ("MeasOut"=w183:T3)  [unwired: 9 in]
            }
            frame 45 {
              n168 = call "meanAllMeaser (SubVI).vi"("mMean"=w185, "MeasIn"=w187) -> ("MeasOut"=w186:T3)  [unwired: 9 in]
            }
            frame 46 {
              n169 = call "meanAllMeaser (SubVI).vi"("mMean"=w188, "MeasIn"=w190) -> ("MeasOut"=w189:T3)  [unwired: 9 in]
            }
            frame 47 {
              n170 = call "meanAllMeaser (SubVI).vi"("mMean"=w191, "MeasIn"=w193) -> ("MeasOut"=w192:T3)  [unwired: 9 in]
            }
            frame 48 {
              n171 = call "meanAllMeaser (SubVI).vi"("mMean"=w194, "MeasIn"=w196) -> ("MeasOut"=w195:T3)  [unwired: 9 in]
            }
            frame 49 {
              n172 = call "meanAllMeaser (SubVI).vi"("mMean"=w197, "MeasIn"=w199) -> ("MeasOut"=w198:T3)  [unwired: 9 in]
            }
            frame 50 {
              n173 = call "meanAllMeaser (SubVI).vi"("mMean"=w200, "MeasIn"=w202) -> ("MeasOut"=w201:T3)  [unwired: 9 in]
            }
            frame 51 {
              n174 = call "meanAllMeaser (SubVI).vi"("mMean"=w203, "MeasIn"=w205) -> ("MeasOut"=w204:T3)  [unwired: 9 in]
            }
            frame 52 {
              n175 = call "meanAllMeaser (SubVI).vi"("mMean"=w206, "MeasIn"=w208) -> ("MeasOut"=w207:T3)  [unwired: 9 in]
            }
            frame 53 {
              n176 = call "meanAllMeaser (SubVI).vi"("mMean"=w209, "MeasIn"=w211) -> ("MeasOut"=w210:T3)  [unwired: 9 in]
            }
            frame 54 {
              n177 = call "meanAllMeaser (SubVI).vi"("mMean"=w212, "MeasIn"=w214) -> ("MeasOut"=w213:T3)  [unwired: 9 in]
            }
            frame 55 {
              n178 = call "meanAllMeaser (SubVI).vi"("mMean"=w215, "MeasIn"=w217) -> ("MeasOut"=w216:T3)  [unwired: 9 in]
            }
            frame 56 {
              n179 = call "meanAllMeaser (SubVI).vi"("mMean"=w218, "MeasIn"=w220) -> ("MeasOut"=w219:T3)  [unwired: 9 in]
            }
            frame 57 {
              n180 = call "meanAllMeaser (SubVI).vi"("mMean"=w221, "MeasIn"=w223) -> ("MeasOut"=w222:T3)  [unwired: 9 in]
            }
            frame 58 {
              n181 = call "meanAllMeaser (SubVI).vi"("mMean"=w224, "MeasIn"=w226) -> ("MeasOut"=w225:T3)  [unwired: 9 in]
            }
            frame 59 {
              n182 = call "meanAllMeaser (SubVI).vi"("mMean"=w227, "MeasIn"=w229) -> ("MeasOut"=w228:T3)  [unwired: 9 in]
            }
            frame 60 {
              n183 = call "meanAllMeaser (SubVI).vi"("mMean"=w230, "MeasIn"=w232) -> ("MeasOut"=w231:T3)  [unwired: 9 in]
            }
            frame 61 {
              n184 = call "meanAllMeaser (SubVI).vi"("mMean"=w233, "MeasIn"=w235) -> ("MeasOut"=w234:T3)  [unwired: 9 in]
            }
            frame 62 {
              n185 = call "meanAllMeaser (SubVI).vi"("mMean"=w236, "MeasIn"=w238) -> ("MeasOut"=w237:T3)  [unwired: 9 in]
            }
            frame 63 {
              n186 = call "meanAllMeaser (SubVI).vi"("mMean"=w239, "MeasIn"=w241) -> ("MeasOut"=w240:T3)  [unwired: 9 in]
            }
            frame 64 {
              n187 = call "meanAllMeaser (SubVI).vi"("mMean"=w242, "MeasIn"=w244) -> ("MeasOut"=w243:T3)  [unwired: 9 in]
            }
            frame 65 {
              n188 = call "meanAllMeaser (SubVI).vi"("mMean"=w245, "MeasIn"=w247) -> ("MeasOut"=w246:T3)  [unwired: 9 in]
            }
            frame 66, Default {
              n189 = call "meanAllMeaser (SubVI).vi"("mMean"=w248, "MeasIn"=w250) -> ("MeasOut"=w249:T3)  [unwired: 9 in]
            }
          }
        }
      }
      "Meas" <- w15
    }
  }
